vi "dy xy calc speed .vi"(4 "DYNAMIC 2":T3(array[cluster]), 6 "DYNAMIC":T3(array[cluster]), 9 "Axis":enum16{"X", "Y", "X+Y"}(ring), 10 "Array 2":T4(array[cluster]), 11 "Data IN":T2={"App State"="", "Connect "=FALSE, "phandle out"=0, "Axis"=[], "S ramp"=30.0, "Acceleration"=100000.0, "Initial Speed"=10.0, "Normal Open / Close"=enum."Close", "Deceleration"=100000.0, "Creep"=30.0, "Speed"=1000.0, "X Axis"={"Operating State"="", "Current Position"=0.0, "Current Speed"=0.0, "Axis State"=0, "Angle"=0.0}, "Y Axis"={"Operating State"="", "Current Position"=0.0, "Current Speed"=0.0, "Axis State"=0, "Angle"=0.0}, "Distance"=0.0, "Direct of movement"=enum."Forward", "Move Method"=enum."Continue", "Move Mode"=enum."Relative", "Angle"=enum."0", "Times"=0, "Start Time"=0.0, "Step Flag"=FALSE, "x  dist"=[], "y dist"=[], "x angle array"=[], "y angle array"=[], "index"=0.0, "big motion angle"=0.0, "big angle"=[], "xy dy speed table"=[], "x dy speed table"=[], "y dy speed table"=[], "x dy time"=[], "y dy time"=[], "xy dy time"=[], "dy Path  "=[]}) -> (2 "dy Path":T1(array[cluster]), 3 "Data out":T2={"App State"="", "Connect "=FALSE, "phandle out"=0, "Axis"=[], "S ramp"=30.0, "Acceleration"=100000.0, "Initial Speed"=10.0, "Normal Open / Close"=enum."Close", "Deceleration"=100000.0, "Creep"=30.0, "Speed"=1000.0, "X Axis"={"Operating State"="", "Current Position"=0.0, "Current Speed"=0.0, "Axis State"=0, "Angle"=0.0}, "Y Axis"={"Operating State"="", "Current Position"=0.0, "Current Speed"=0.0, "Axis State"=0, "Angle"=0.0}, "Distance"=0.0, "Direct of movement"=enum."Forward", "Move Method"=enum."Continue", "Move Mode"=enum."Relative", "Angle"=enum."0", "Times"=0, "Start Time"=0.0, "Step Flag"=FALSE, "x  dist"=[], "y dist"=[], "x angle array"=[], "y angle array"=[], "index"=0.0, "big motion angle"=0.0, "big angle"=[], "xy dy speed table"=[], "x dy speed table"=[], "y dy speed table"=[], "x dy time"=[], "y dy time"=[], "xy dy time"=[], "dy Path  "=[]})   [LabVIEW 2015]
uses:
  Typedef/Data2.ctl
panel:
  in  "Speed":dbl=1.0 format="%#_13g"
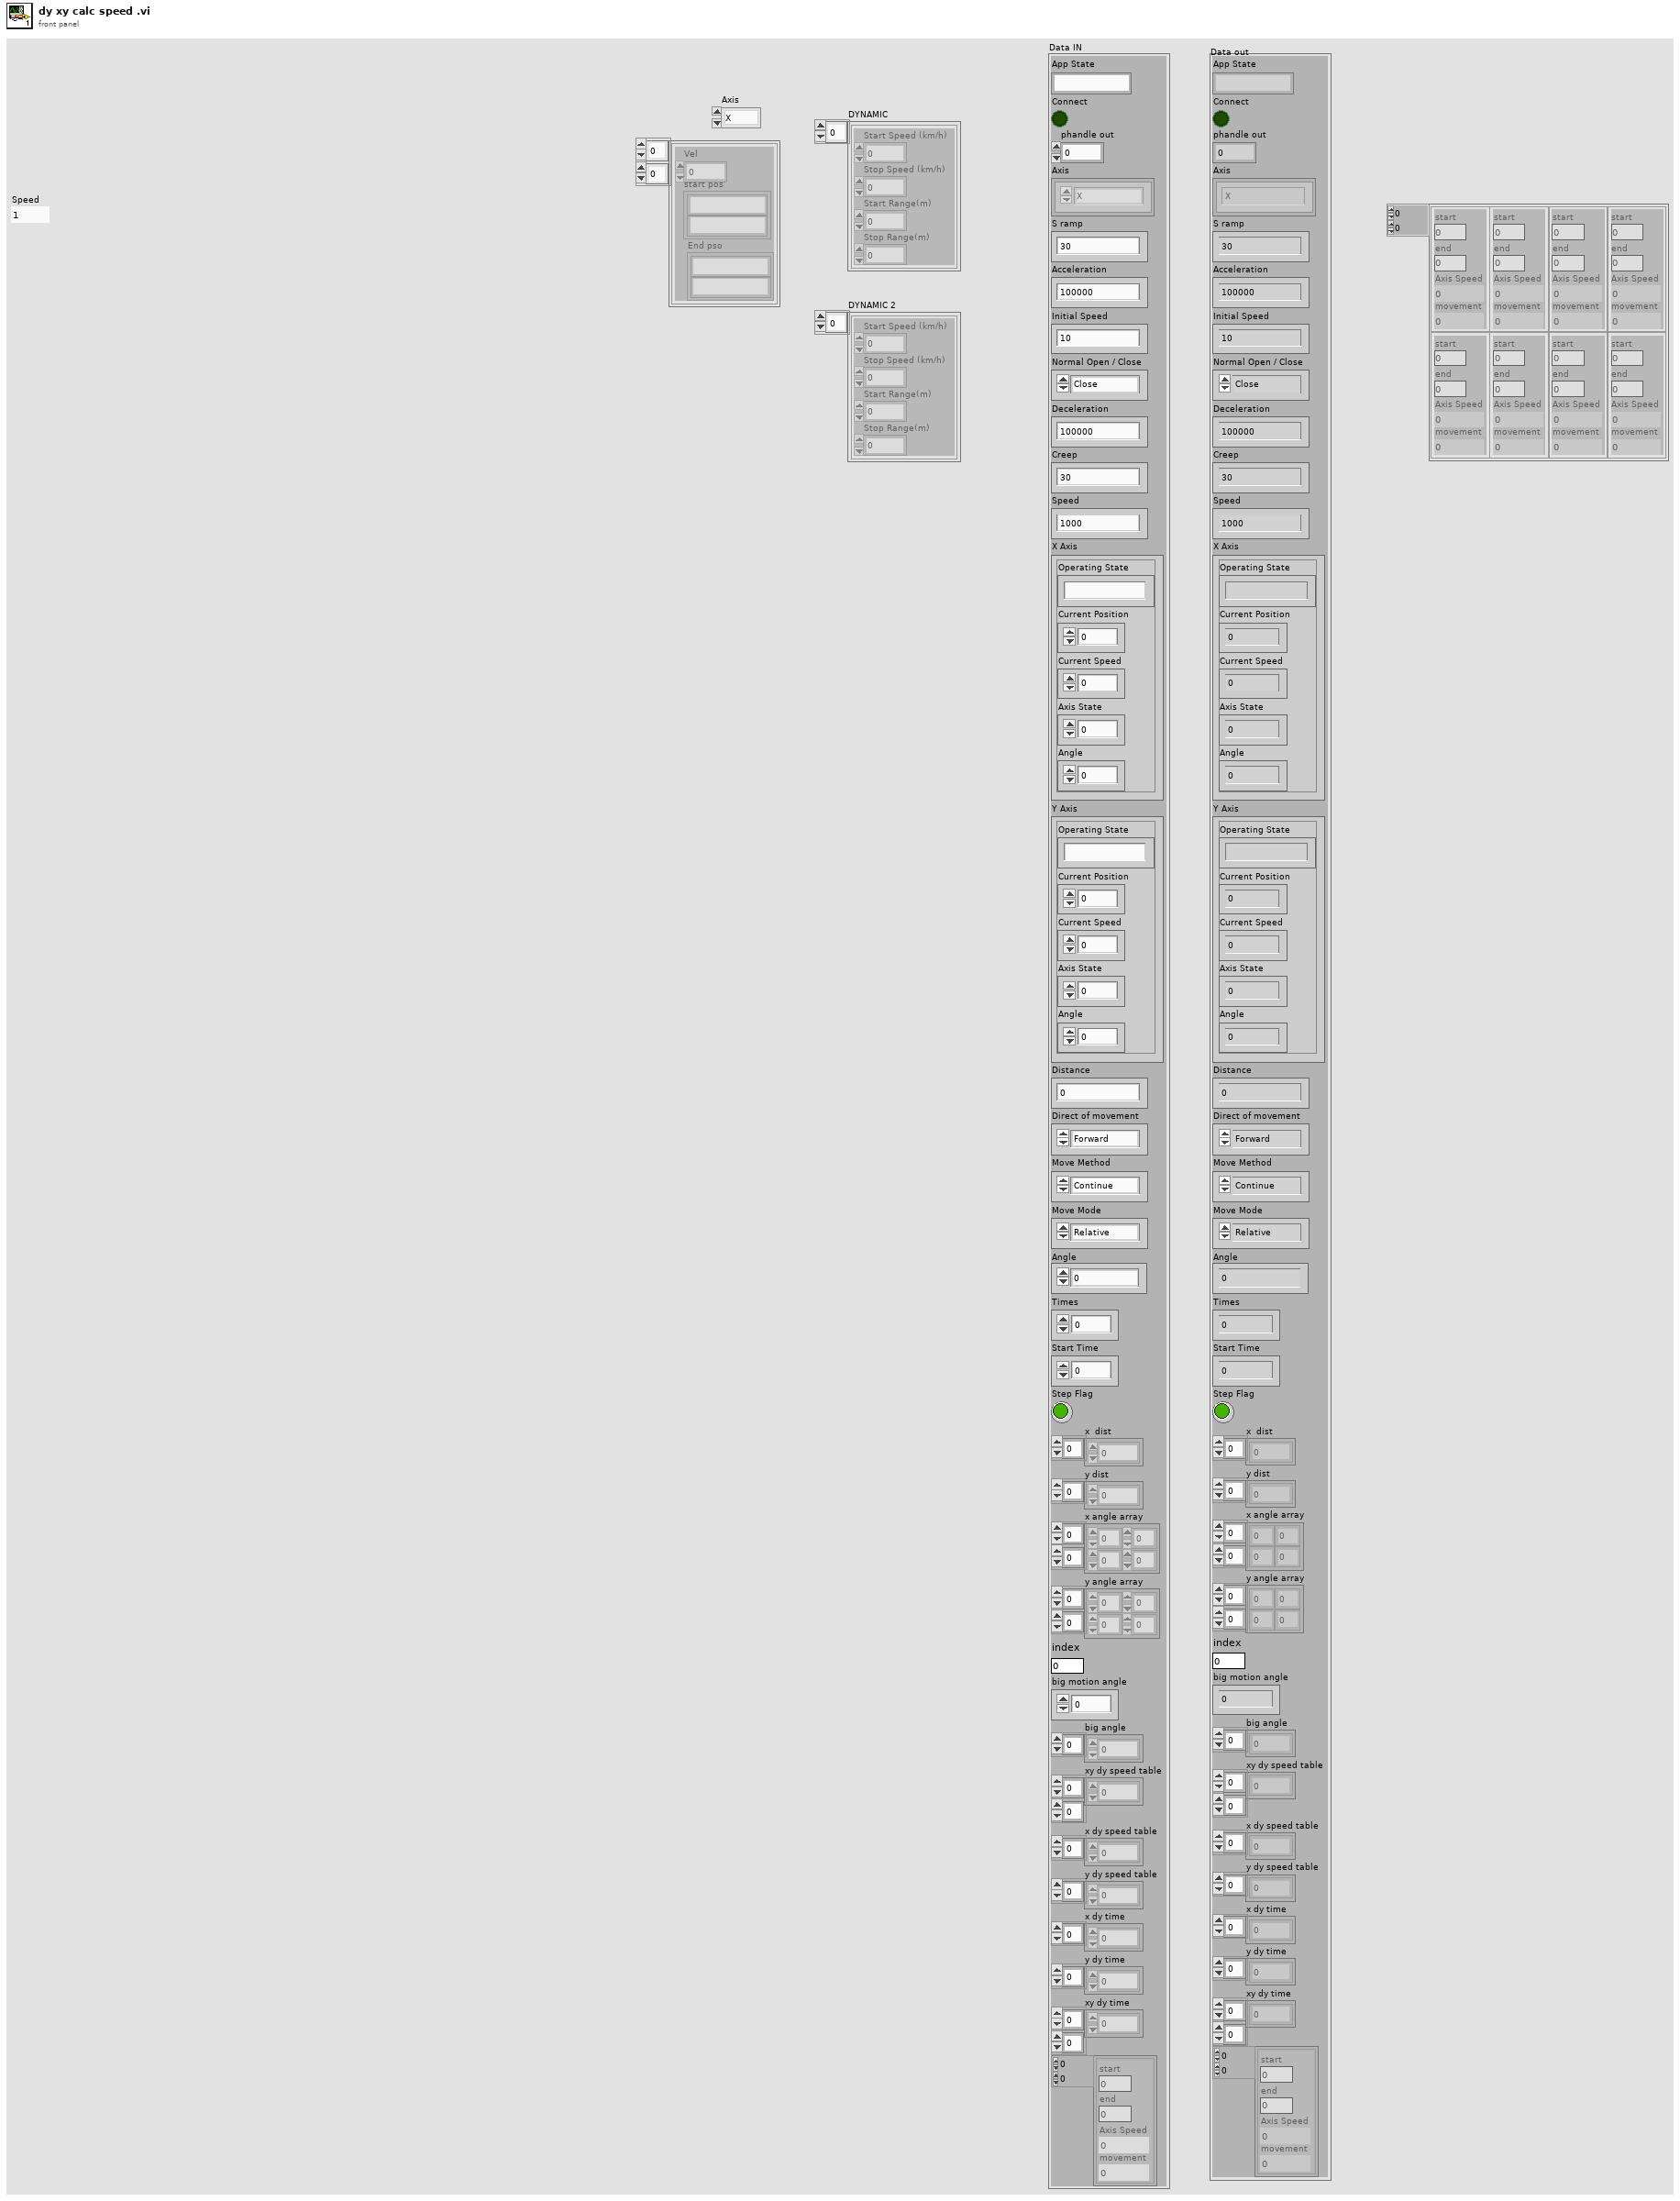
[diagram p1: front panel]
types:
  T1 = cluster{"end":dbl, "start":dbl, "Axis Speed":dbl, "movement":dbl}[][]
  T2 = typedef "Data2.ctl" = cluster{"App State":string, "Connect ":bool, "phandle out":u32, "Axis":enum16{"X", "Y", "X+Y"}[], "S ramp":dbl, "Acceleration":dbl, "Initial Speed":dbl, "Normal Open / Close":enum16{"Open", "Close"}, "Deceleration":dbl, "Creep":dbl, "Speed":dbl, "X Axis":cluster{"Operating State":string, "Current Position":dbl, "Current Speed":dbl, "Axis State":i32, "Angle":dbl}, "Y Axis":cluster{"Operating State":string, "Current Position":dbl, "Current Speed":dbl, "Axis State":i32, "Angle":dbl}, "Distance":dbl, "Direct of movement":enum16{"Forward", "Backward"}, "Move Method":enum16{"Continue", "Inching"}, "Move Mode":enum16{"Relative", "Absolute"}, "Angle":enum32{"0", "1", "10", "30", "34", "60", "90", "180", "-1", "-10"}, "Times":i32, "Start Time":dbl, "Step Flag":bool, "x  dist":dbl[], "y dist":dbl[], "x angle array":i32[][], "y angle array":i32[][], "index":dbl, "big motion angle":dbl, "big angle":dbl[], "xy dy speed table":dbl[][], "x dy speed table":dbl[], "y dy speed table":dbl[], "x dy time":dbl[], "y dy time":dbl[], "xy dy time":dbl[][], "dy Path  ":cluster{"end":dbl, "start":dbl, "Axis Speed":dbl, "movement":dbl}[][]}
  T3 = cluster{"Start Speed (km/h)":dbl, "Stop Speed (km/h) ":dbl, "Start Range(m)":dbl, "Stop Range(m)":dbl}[]
  T4 = cluster{"Vel":dbl, "start pos":cluster{string, string}, "End pso":cluster{string, string}}[][]
  T5 = cluster{"end":dbl, "start":dbl, "Axis Speed":dbl, "movement":dbl}
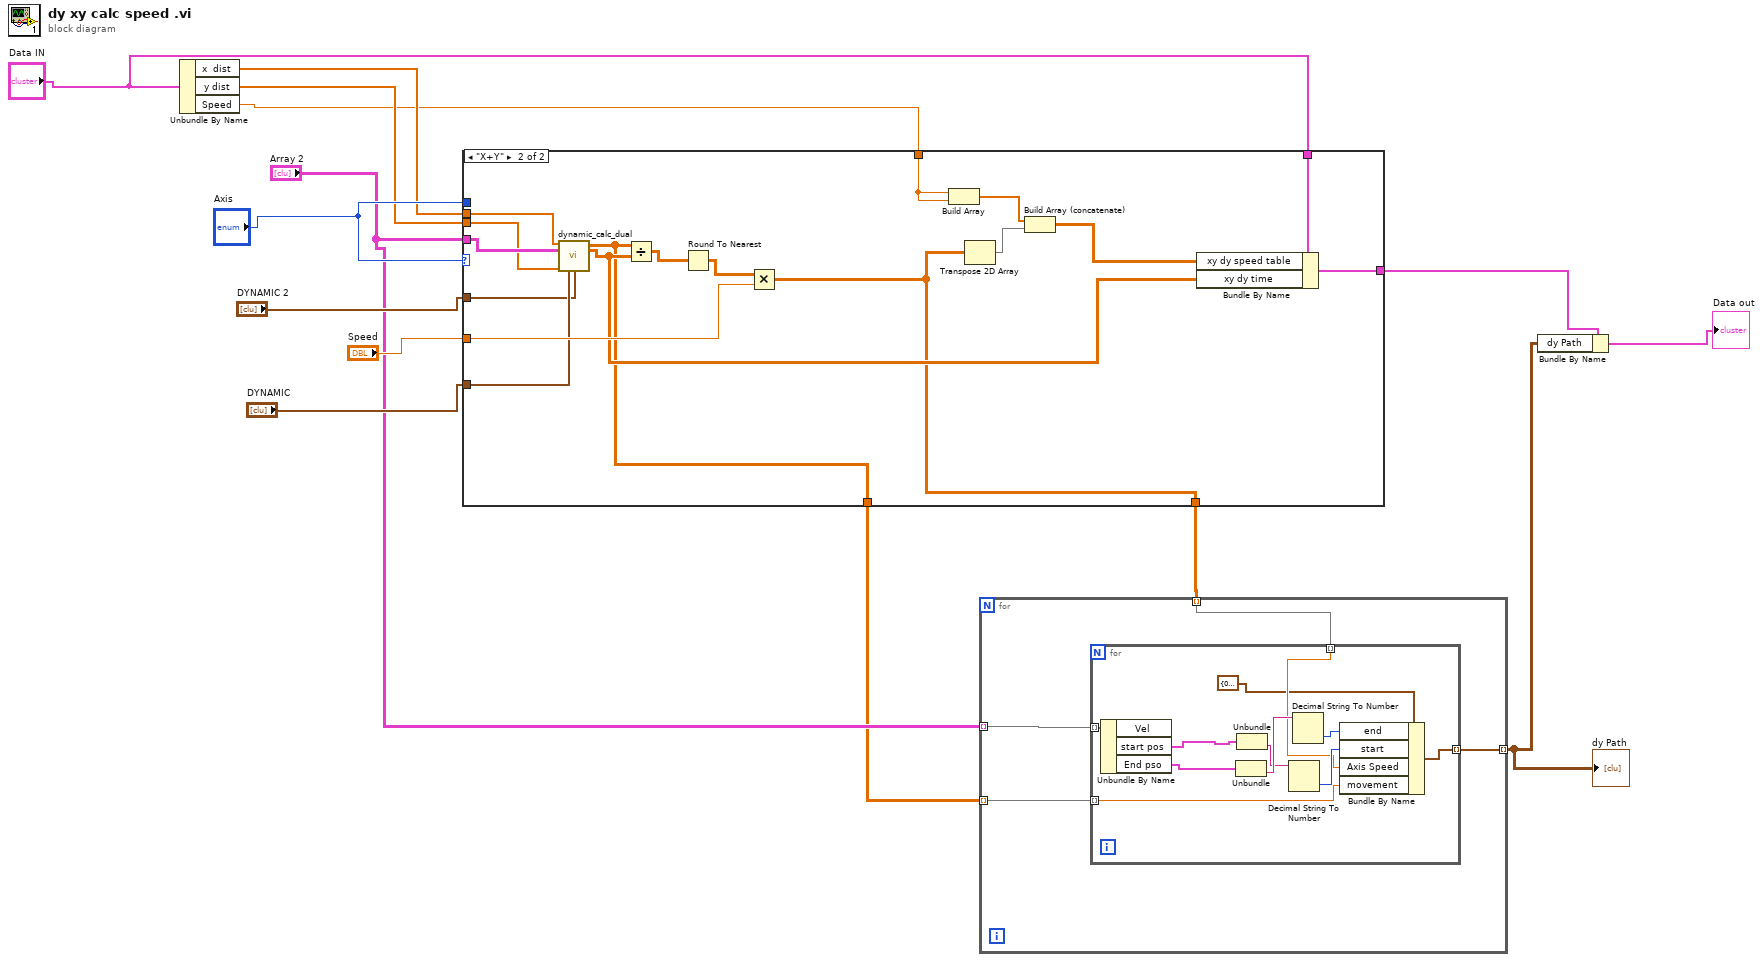
[diagram p0: block diagram]
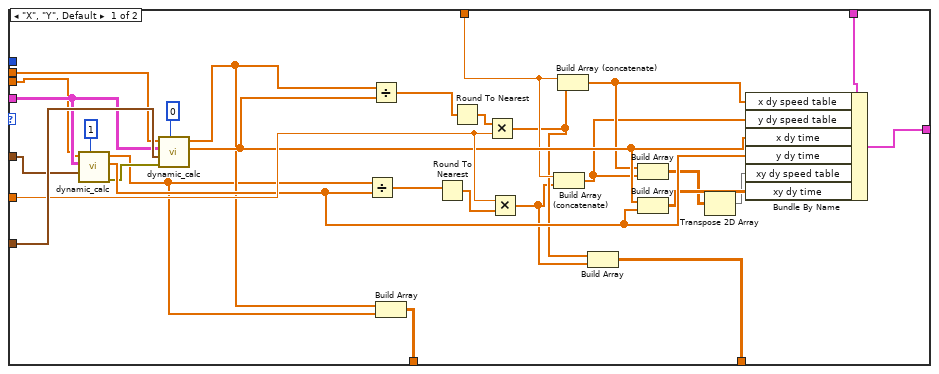
[diagram p2: hidden frame]
diagram:
  n1 = Unbundle By Name("Data IN") -> ("x  dist"=w12:dbl[], "y dist"=w11:dbl[], "Speed"=w10:dbl)
  n2 = case shown="\"X+Y\"" "Axis" {
    tunnel: "DYNAMIC 2" -> [w36 w46]
    tunnel: "Array 2" -> [w37 w60]
    tunnel: w12 -> [w23 w59]
    tunnel: w11 -> [w22 w58]
    tunnel: "Axis" -> [_ _]
    tunnel: "Speed" -> [w33 w55]
    tunnel: "DYNAMIC" -> [w41 w47]
    tunnel: w10 -> [w26 w54]
    tunnel: "Data IN" -> [w39 w51]
    tunnel: [w38 w50] -> w4
    tunnel: [w18 w45] -> w5
    tunnel: [w15 w44] -> w2
    frame "X", "Y", Default {
      n3 = call "dynamic_calc.vi"("index (row)"=1, "DYNAMIC"=w36, "Array 2"=w37, "x  dist"=w22) -> ("error constant 2"=w24:errorcluster, "time"=w30:dbl[], "Array"=w16:dbl[])  [unwired: 5 in]
      n4 = call "dynamic_calc.vi"("index (row)"=0, "error constant"=w24, "DYNAMIC"=w41, "Array 2"=w37, "x  dist"=w23) -> ("time"=w31:dbl[], "Array"=w17:dbl[])  [unwired: 4 in, 1 out]
      n5 = Divide(x=w16, y=w30) -> (x/y=w34:dbl[])
      n6 = Divide(x=w17, y=w31) -> (x/y=w40:dbl[])
      n7 = Build Array(w17, w16) -> (w15:dbl[][])
      n8 = Round To Nearest(number=w34) -> (nearest integer value=w32:dbl[])
      n9 = Round To Nearest(number=w40) -> (nearest integer value=w43:dbl[])
      n10 = Multiply(x=w43, y=w33) -> (x*y=w20:dbl[])
      n11 = Multiply(x=w33, y=w32) -> (x*y=w19:dbl[])
      n12 = Build Array (concatenate)(w26, w19) -> (w27:dbl[])
      n13 = Build Array (concatenate)(w26, w20) -> (w28:dbl[])
      n14 = Build Array(w20, w19) -> (w18:dbl[][])
      n15 = Build Array(w28, w27) -> (w25:dbl[][])
      n16 = Build Array(w31, w30) -> (w29:dbl[][])
      n17 = Transpose 2D Array(2D array=w25) -> (transposed array=w21:dbl[][])
      n18 = Bundle By Name(cluster=w39, "x dy speed table"=w28, "y dy speed table"=w27, "x dy time"=w31, "y dy time"=w30, "xy dy speed table"=w21, "xy dy time"=w29) -> (w38:T2)
    }
    frame "X+Y" {
      n19 = call "dynamic_calc_dual.vi"("x  dist"=w59, "Array 2"=w60, "y  dist"=w58, "DYNAMIC"=w47, "DYNAMIC 2"=w46) -> ("dist"=w44:dbl[][], "time"=w52:dbl[][])  [unwired: 9 in]
      n20 = Divide(x=w44, y=w52) -> (x/y=w57:dbl[][])
      n21 = Round To Nearest(number=w57) -> (nearest integer value=w56:dbl[][])
      n22 = Multiply(x=w56, y=w55) -> (x*y=w45:dbl[][])
      n23 = Build Array(w54, w54) -> (w53:dbl[])
      n24 = Transpose 2D Array(2D array=w45) -> (transposed array=w48:dbl[][])
      n25 = Build Array (concatenate)(w53, w48) -> (w49:dbl[][])
      n26 = Bundle By Name(cluster=w51, "xy dy speed table"=w49, "xy dy time"=w52) -> (w50:T2)
    }
  }
  n27 = for {
    tunnel: "Array 2" -> [w64] mode=indexing
    tunnel: w5 -> [w63] mode=indexing
    tunnel: [w62] -> w1 mode=indexing
    tunnel: w2 -> [w61] mode=indexing
    n28 = for {
      tunnel: w64 -> [w75] mode=indexing
      tunnel: w63 -> [w68] mode=indexing
      tunnel: [w67] -> w62 mode=indexing
      tunnel: w61 -> [w65] mode=indexing
      n29 = Unbundle By Name(w75) -> ("start pos"=w74:cluster{string, string}, "End pso"=w73:cluster{string, string})  [unwired: 1 out]
      n30 = Unbundle(w73) -> (w72:string)  [unwired: 1 out]
      n31 = Unbundle(w74) -> (w71:string)  [unwired: 1 out]
      n32 = Decimal String To Number(string=w71) -> (number=w69:i32)  [unwired: 2 in, 1 out]
      n33 = Decimal String To Number(string=w72) -> (number=w70:i32)  [unwired: 2 in, 1 out]
      n34 = Bundle By Name(cluster=T5 {"end"=0.0, "start"=0.0, "Axis Speed"=0.0, "movement"=0.0} ("dy Path   2"), "end"=w70, "start"=w69, "Axis Speed"=w68, "movement"=w65) -> (w67:T5)
    }
  }
  "dy Path" <- w1
  n35 = Bundle By Name(cluster=w4, "dy Path"=w1) -> (→"Data out":T2)
